vi "ADV PID 2.vi"(9 "Time":dbl, 10 "SP-SetPoint in":dbl, 11 "PV-Measurement in":dbl) -> (3 "CO-ControlOutput":dbl)   [LabVIEW 2020]
uses:
  <vilib>/Rock Robotics/WPI/ThirdParty/JAS_Junk/TrajLib/PIDController_AtSetpoint.vi
  <vilib>/Rock Robotics/WPI/ThirdParty/JAS_Junk/TrajLib/PIDController_SetPIDF.vi
  <vilib>/Rock Robotics/WPI/ThirdParty/JAS_Junk/TrajLib/PIDController_SetDerivativeFilter.vi
  <vilib>/Rock Robotics/WPI/ThirdParty/JAS_Junk/TrajLib/PIDController_SetIntegratorRange.vi
  <vilib>/Rock Robotics/WPI/ThirdParty/JAS_Junk/TrajLib/PIDController_SetTolerancePandV.vi
  <vilib>/Rock Robotics/WPI/ThirdParty/JAS_Junk/TrajLib/PIDController_DisableContinousInput.vi
  <vilib>/Rock Robotics/WPI/ThirdParty/JAS_Junk/TrajLib/PIDController_EnableContinousInput.vi
  <vilib>/Rock Robotics/WPI/ThirdParty/JAS_Junk/TrajLib/PIDController_Reset.vi
  <vilib>/Rock Robotics/WPI/ThirdParty/JAS_Junk/TrajLib/PIDController_New.vi
  <vilib>/Rock Robotics/WPI/ThirdParty/JAS_Junk/TrajLib/PIDController_SetOutputLimits.vi
  <vilib>/Rock Robotics/WPI/ThirdParty/JAS_Junk/TrajLib/PIDController_NewPeriod.vi
  <vilib>/Rock Robotics/SystemInterfaces/NetworkCommunication/NetComm_UsageReport_report.vi
  <vilib>/Rock Robotics/WPI/ThirdParty/JAS_Junk/TrajLib/Util_LibraryGlobals.vi
  <vilib>/Rock Robotics/WPI/ThirdParty/JAS_Junk/TrajLib/PIDController_AdvCalculate_FF_Sp_Pv.vi
  <vilib>/Rock Robotics/WPI/ThirdParty/JAS_Junk/TrajLib/Trajectory_Library.lvlib
panel:
  in  "Kd":dbl format="%#_13g"
  in  "Ki":dbl format="%#_13g"
  in  "Kp":dbl=0.5 format="%#_13g"
  in  "Kf":dbl format="%#_13g"
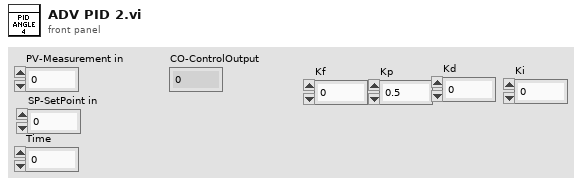
[diagram p1: front panel]
types:
  T1 = typedef "Trajectory_Library.lvlib/PID_ADV_LIMITS.ctl" = cluster{"MaxInput":dbl, "MinInput":dbl, "Continuous":bool, "MaxOutput":dbl, "MinOutput":dbl}
  T2 = typedef "Trajectory_Library.lvlib/PID_ADV_TUNING.ctl" = cluster{"Kf":dbl, "Kp":dbl, "Ki":dbl, "Kd":dbl, "MaximumIntegral":dbl, "MinimumIntegral":dbl, "Filter Derivative":bool}
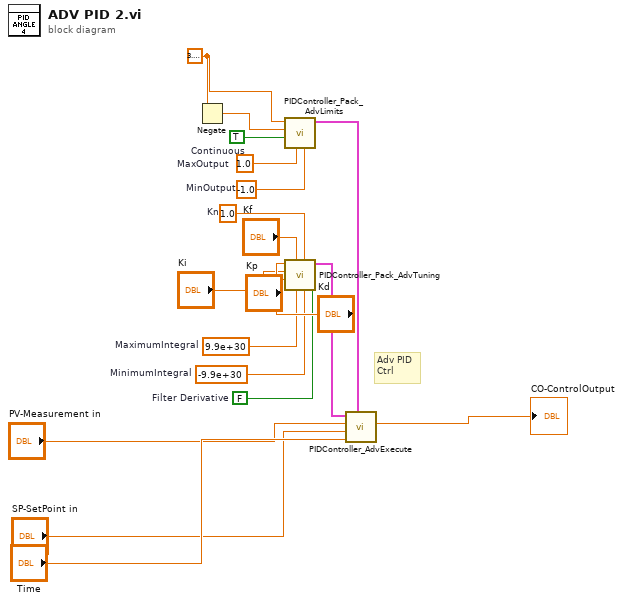
[diagram p0: block diagram]
diagram:
  w1 = 3.141592653589793
  w18 = 1.0  # Kn
  w13 = 9.9e+30  # MaximumIntegral
  w12 = -9.9e+30  # MinimumIntegral
  w11 = FALSE  # Filter Derivative
  w9 = TRUE  # Continuous
  w8 = 1.0  # MaxOutput
  w10 = -1.0  # MinOutput
  # "Adv PID\nCtrl"
  n1 = Negate(x=w1) -> (-x=w2:dbl)
  n2 = call <vilib>:"PIDController_Pack_AdvLimits.vi"("MinOutput"=w10, "MaxOutput"=w8, "Continuous"=w9, "MinInput"=w2, "MaxInput"=w1) -> ("Adv PID Limits"=w6:T1)  [unwired: 6 in]
  n3 = call <vilib>:"PIDController_Pack_AdvTuning.vi"("Filter Derivative"=w11, "MinimumIntegral"=w12, "Kn"=w18, "MaximumIntegral"=w13, "Kf"="Kf", "Kd"="Kd", "Ki"="Ki", "Kp"="Kp") -> ("Adv PID Tuning"=w7:T2)  [unwired: 3 in]
  n4 = call <vilib>:"PIDController_AdvExecute.vi"("Time"="Time", "Adv PID Limits"=w6, "SP-SetPoint"="SP-SetPoint in", "PV-Measurement"="PV-Measurement in", "Adv PID Tuning"=w7) -> ("CO-ControlOutput"=→"CO-ControlOutput":dbl)  [unwired: 4 in, 2 out]
